vi "Command Reply.vi"(8 "error in":errorcluster, 10 "cmd successful":bool, 11 "CMD in":refnum<class "Command.lvclass">) -> (0 "error out":errorcluster, 3 "CMD out":refnum<class "Command.lvclass">)   [LabVIEW 2016, in "Command.lvclass"]
doc: "Provide a manner to broadcast command success from target. This relies on the caller setting up the queue for the response. If no queue is present, then the boolean value is not sent."
uses:
  Command.lvclass
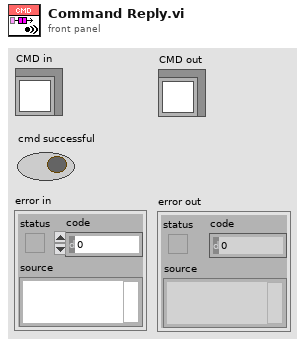
[diagram p1: front panel]
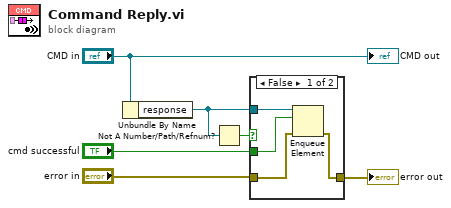
[diagram p0: block diagram]
diagram:
  n1 = Unbundle By Name("CMD in") -> ("response"=w4:refnum<queue>)
  n2 = Not A Number/Path/Refnum?(number/path/refnum=w4) -> (NaN/Path/Refnum?=w5:bool)
  n3 = case shown="False" w5 {
    tunnel: w4 -> [w10 _]
    tunnel: "cmd successful" -> [w9 _]
    tunnel: "error in" -> [w8 w11]
    tunnel: [w7 w11] -> w1
    frame False {
      n4 = Enqueue Element(queue=w10, element=w9, error in (no error)=w8) -> (error out=w7:errorcluster)  [unwired: 1 in, 2 out]
    }
    frame True {
    }
  }
  "error out" <- w1
  "CMD out" <- "CMD in"
